vi "Initialize.vi"(8 "error in (no error)":errorcluster, 9 "ID Query (True)":bool=TRUE, 10 "Serial Configuration":T1={"Baud Rate"=9600, "Parity"=0, "Data Bits"=7, "Stop Bits"=10, "Flow Control"=0} {"Flow Control" items=["None", "XON/XOFF", "RTS/CTS", "XON/XOFF & RTS/CTS", "DTR/DSR", "XON/XOFF & DTR/DSR"]; "Stop Bits" items=["1.0"=10, "1.5"=15, "2.0"=20]; "Data Bits" items=["7"=7, "8"=8]; "Parity" items=["None", "Odd", "Even", "Mark", "Space"]; "Baud Rate" items=["300"=300, "600"=600, "1200"=1200, "2400"=2400, "4800"=4800, "9600"=9600, "19200"=19200]}, 11 "VISA resource name":refnum<visa-resource-name>) -> (0 "error out":errorcluster, 3 "VISA resource name out":refnum<visa-resource-name>)   [LabVIEW 2017, in "RadWag balances and scales.lvlib"]
doc: "Establishes communication with the instrument and optionally performs an instrument identification query and/or an instrument reset. It also places the instrument in a default state needed for other instrument driver operations. Therefore, call this VI before calling other instrument driver VIs for this instrument. Generally, you need to call the <b>Initialize</b> VI only once at the beginning of an application.\n\n<b>Notes</b>\nMake sure, that the transmission parameters (baud rate, parity, etc.) are configured indentically as in your balance.\nIf some parameters are not configurable on balance, use the default values of this VI."
uses:
  <instrlib>/Prev/RadWag Continuous Read Folder/RadWag balances and scales.lvlib
panel:
  # "(c) 2014 Przemysłowy Instytut Automatyki i Pomiarów PIAP.  ALL RIGHTS RESERVED."
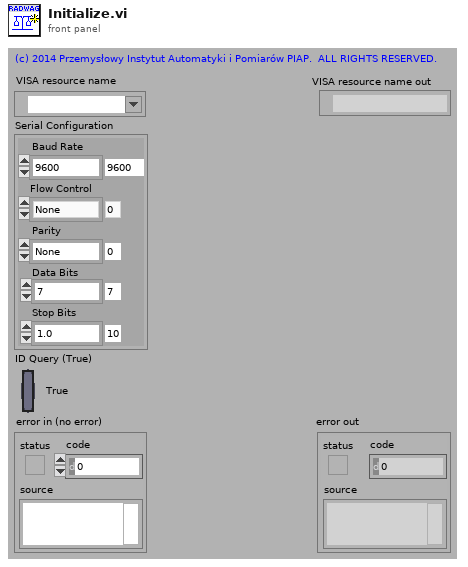
[diagram p1: front panel]
types:
  T1 = cluster{"Baud Rate":u32, "Parity":u16, "Data Bits":u16, "Stop Bits":u16, "Flow Control":u16}
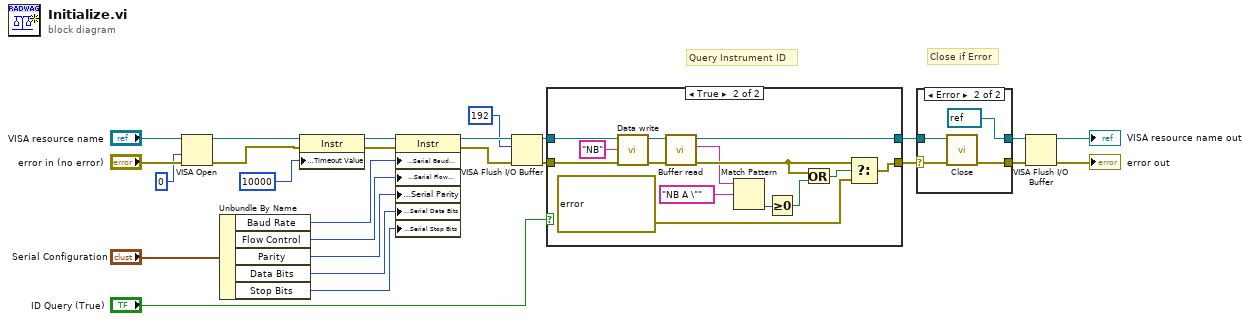
[diagram p0: block diagram]
diagram:
  # "Close if Error"
  # "Query Instrument ID"
  n1 = VISA Open(access mode=u32 0, error in (no error)="error in (no error)", VISA resource name="VISA resource name") -> (VISA resource name=w2:refnum<visa-resource-name>, error out=w1:errorcluster)  [unwired: 2 in]
  n2 = Unbundle By Name("Serial Configuration") -> ("Baud Rate"=w11:u32, "Flow Control"=w8:u16, "Parity"=w9:u16, "Data Bits"=w10:u16, "Stop Bits"=w7:u16)
  n3 = property class="Instr"(reference=w2, error in=w1, "General Settings:Timeout Value"=u32 10000) -> (reference out=w22:refnum<visa-resource-name>, error out=w21:errorcluster)
  n4 = property class="Instr"(reference=w22, error in=w21, "Serial Settings:Serial Baud Rate"=w11, "Serial Settings:Serial Flow Control"=w8, "Serial Settings:Serial Parity"=w9, "Serial Settings:Serial Data Bits"=w10, "Serial Settings:Serial Stop Bits"=w7) -> (reference out=w13:refnum<visa-resource-name>, error out=w15:errorcluster)
  n5 = VISA Flush I/O Buffer(VISA resource name=w13, mask (16)=u16 192, error in (no error)=w15) -> (VISA resource name out=w16:refnum<visa-resource-name>, error out=w14:errorcluster)
  n6 = case shown="True" "ID Query (True)" {
    tunnel: [w27 w42] -> w17
    tunnel: [w28 w34] -> w18
    tunnel: w16 -> [w28 w30]
    tunnel: w14 -> [w27 w31]
    frame False {
    }
    frame True {
      n7 = call <instrlib>:"Data write.vi"("error in (no error)"=w31, "ID"="NB", "VISA resource name"=w30) -> ("error out"=w36:errorcluster, "VISA resource name out"=w35:refnum<visa-resource-name>)  [unwired: 7 in]
      n8 = call <instrlib>:"Buffer read.vi"("error in (no error)"=w36, "VISA resource name"=w35) -> ("error out"=w33:errorcluster, "Received String"=w32:string, "VISA resource name out"=w34:refnum<visa-resource-name>)  [unwired: 7 in]
      n9 = Match Pattern(string=w32, regular expression="NB A \"") -> (offset past match=w40:i32)  [unwired: 1 in, 3 out]
      n10 = Greater Or Equal To 0?(x=w40) -> (x >= 0?=w39:bool)
      n11 = Or(x=w33, y=w39) -> (x .or. y?=w38:bool)
      n12 = Select(t=w33, s=w38, f=errorcluster {"status"=TRUE, "code"=-1074003951, "source"="The ID Query failed.  This may mean that you selected the wrong instrument or your instrument did not respond.  You may also be using a model that is not officially supported by this driver.  If you are sure that you have selected the correct instrument and it is responding, try disabling the ID Query."} ("error constant")) -> (s? t:f=w42:errorcluster)
    }
  }
  n13 = case shown="Error" w17 {
    selector: w17 -> [w43 w46]
    tunnel: w18 -> [w44 w47]
    tunnel: [w44 refnum<visa-resource-name> refnum ("VISA resource name out")] -> w6
    tunnel: [w43 w45] -> w5
    frame No Error {
    }
    frame Error {
      n14 = call <instrlib>:"Close.vi"("error in (no error)"=w46, "VISA resource name"=w47) -> ("error out"=w45:errorcluster)  [unwired: 9 in]
    }
  }
  n15 = VISA Flush I/O Buffer(VISA resource name=w6, error in (no error)=w5) -> (VISA resource name out=→"VISA resource name out":refnum<visa-resource-name>, error out=→"error out":errorcluster)  [unwired: 1 in]
